vi "LoadClassExecutionInfo.vi"(1 "class in":refnum<class>, 5 "error in (no error)":errorcluster) -> (15 "ClassExecutionInfo":T1, 19 "error out":errorcluster)   [LabVIEW 2018, in "Executer.lvclass"]
uses:
  Executer.lvclass
  typedefs/ClassExecutionInfo.ctl
  typedefs/MethodExecutionInfo.ctl
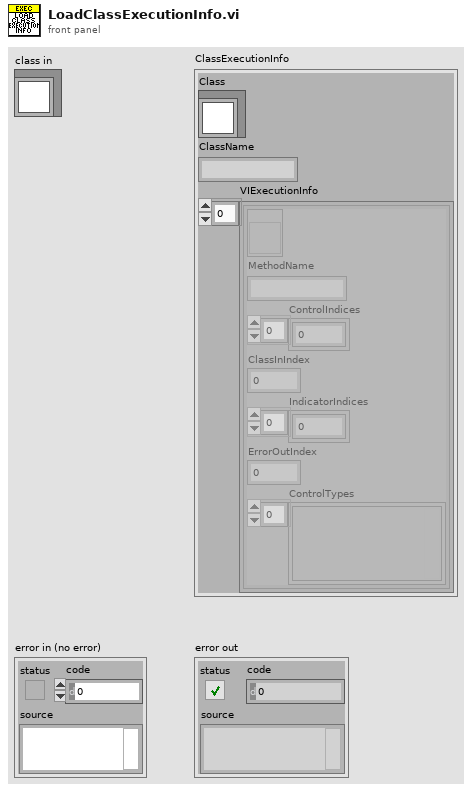
[diagram p1: front panel]
types:
  T1 = typedef "Executer.lvclass/ClassExecutionInfo.ctl" = cluster{"Class":refnum<class>, "ClassName":string, "VIExecutionInfo":T2[]}
  T2 = typedef "Executer.lvclass/MethodExecutionInfo.ctl" = cluster{"viRef":refnum<vi>, "MethodName":string, "ControlIndices":i32[], "ClassInIndex":i32, "IndicatorIndices":i32[], "ErrorOutIndex":i32, "ControlTypes":variant[]}
  T3 = enum32{"invalid scope", "public", "private", "protected", "community"}
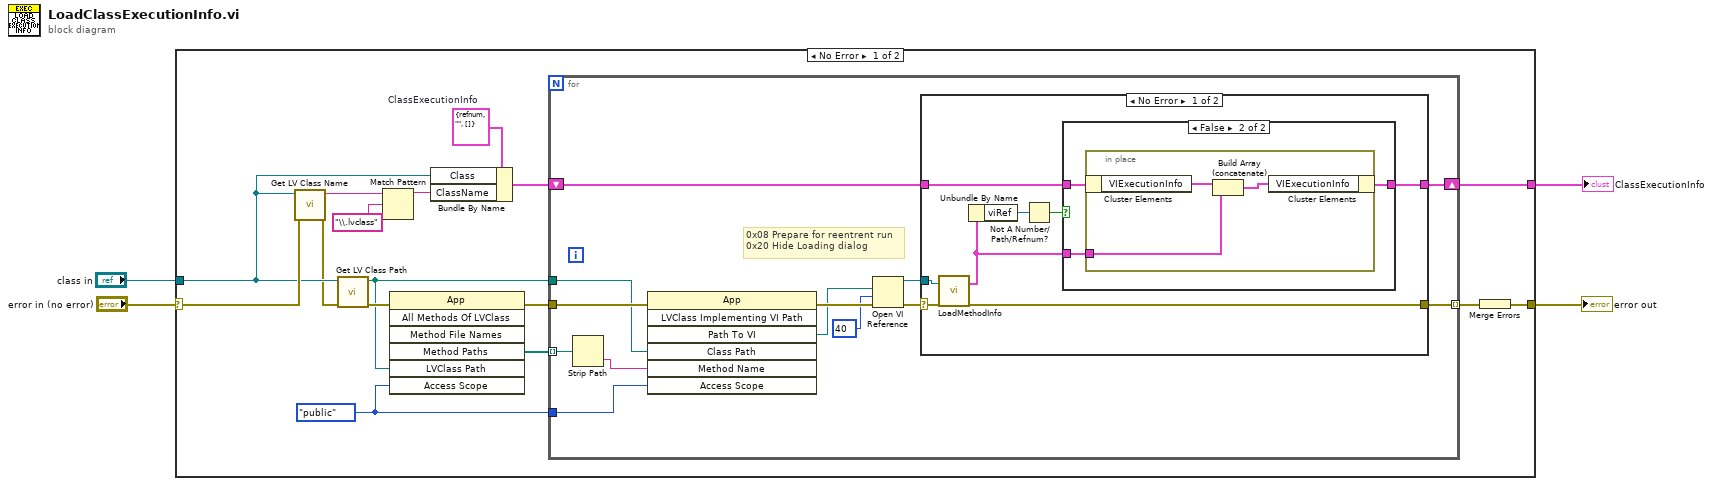
[diagram p0: block diagram]
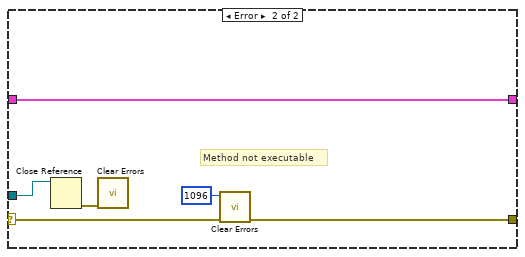
[diagram p3: hidden frame]
diagram:
  n1 = case shown="No Error" "error in (no error)" {
    selector: "error in (no error)" -> [w18 w55]
    tunnel: [w19 w55] -> w3
    tunnel: "class in" -> [w17 _]
    tunnel: [w16 _] -> w1
    frame No Error {
      w10 = T1 {"Class"=refnum, "ClassName"="", "VIExecutionInfo"=[]}  # ClassExecutionInfo
      w15 = T3."public" ("Access Scope")
      n2 = call <vilib>:"Get LV Class Name.vi"("error in (no error)"=w18, "object"=w17) -> ("error out"=w11:errorcluster, "class name"=w6:string)  [unwired: 8 in]
      n3 = call <vilib>:"Get LV Class Path.vi"("error in (no error)"=w11, "object"=w17) -> ("error out"=w12:errorcluster, "class path"=w5:path)  [unwired: 8 in]
      n4 = Match Pattern(string=w6, regular expression="\\.lvclass") -> (before substring=w7:string)  [unwired: 1 in, 3 out]
      n5 = invoke class="App" method="All Methods Of LVClass"(error in=w12, "LVClass Path"=w5, "Access Scope"=w15) -> (error out=w13:errorcluster, "Method Paths"=w14:path[])  [unwired: 4 in, 5 out]
      n6 = Bundle By Name(cluster=w10, "Class"=w17, "ClassName"=w7) -> (w9:T1)
      n7 = for {
        tunnel: w5 -> [w25]
        tunnel: w15 -> [w33]
        tunnel: w14 -> [w24] mode=indexing
        tunnel: w13 -> [w32]
        tunnel: [w31] -> w20 mode=indexing
        shift-right: [w29] -> w16
        shift-left: w9 -> [w30]
        # "0x08 Prepare for reentrent run\n0x20 Hide Loading dialog"
        n8 = Strip Path(path=w24) -> (name=w22:string)  [unwired: 1 out]
        n9 = invoke class="App" method="LVClass Implementing VI Path"(error in=w32, "Class Path"=w25, "Method Name"=w22, "Access Scope"=w33) -> (error out=w27:errorcluster, "Path To VI"=w23:path)  [unwired: 3 in, 5 out]
        n10 = Open VI Reference(vi path=w23, options=40, error in (no error)=w27) -> (vi reference=w28:refnum<vi>, error out=w26:errorcluster)  [unwired: 3 in]
        n11 = case shown="No Error" w26 {
          selector: w26 -> [w35 w50]
          tunnel: [w34 w54] -> w31
          tunnel: w28 -> [w41 w53]
          tunnel: w30 -> [w39 w51]
          tunnel: [w38 w51] -> w29
          frame No Error {
            n12 = call "LoadMethodInfo.vi"("ViRef"=w41, "error in (no error)"=w35) -> ("ExecutionInfo"=w37:T2, "error out"=w34:errorcluster)  [unwired: 15 in, 1 out]
            n13 = Unbundle By Name(w37) -> ("viRef"=w40:refnum<vi>)
            n14 = Not A Number/Path/Refnum?(number/path/refnum=w40) -> (NaN/Path/Refnum?=w36:bool)
            n15 = case shown="False" w36 {
              tunnel: w37 -> [_ w43]
              tunnel: w39 -> [w42 w45]
              tunnel: [w42 w44] -> w38
              frame True {
              }
              frame False {
                n16 = in-place {
                  in-place-border: w43 -> [w46]
                  n17 = in-place-cluster #1(w45) -> ("VIExecutionInfo"=w48:T2[])
                  n18 = Build Array (concatenate)(w48, w46) -> (w47:T2[])
                  n19 = in-place-cluster #1("VIExecutionInfo"=w47) -> (w44:T1)
                }
              }
            }
          }
          frame Error {
            # "Method not executable"
            n20 = Close Reference(reference=w53) -> (error out=w49:errorcluster)  [unwired: 1 in]
            n21 = call <vilib>:"Clear Errors.vi"("error in (no error)"=w49) -> ()  [unwired: 5 in, 2 out]
            n22 = call <vilib>:"Clear Errors.vi"("error in (no error)"=w50, "specific error code to clear (0: all)"=1096) -> ("error out"=w54:errorcluster)  [unwired: 4 in, 1 out]
          }
        }
      }
      n23 = Merge Errors(w20) -> (w19:errorcluster)
    }
    frame Error {
    }
  }
  "error out" <- w3
  "ClassExecutionInfo" <- w1
